vi "main(Test DQMH modules).vi"() -> ()   [LabVIEW 2018, in "Application.lvlib"] (continued)
          n6544 = Unbundle By Name(w14061) -> ("command"=w14060:string, "data"=w14059:variant)
          n6545 = call "App enquece.vi"("command data"=w14059, "command"=w14060, "queue in"=w14062) -> ("error out"=w14058:errorcluster)  [unwired: 7 in, 1 out]
        }
        n6546 = Merge Errors(w13977, w13976) -> (w13975:errorcluster)
      }
      frame "Test DRV 43A" {
        w14066 = 43 ("DUT index(0-59)")
        n6547 = disable-structure shown="LOGGING==TRUE" {
          disable-tunnel: w14071 -> [w14154 _]
          frame condition #0 (active) {
            n6548 = Empty String/Path?(string/path=w14154) -> (empty?=w14156:bool)
            n6549 = Select(t="Quece timeout", s=w14156, f=w14154) -> (s? t:f=w14153:string)
            n6550 = call "string log (SubVI).vi"("state Name"=w14153) -> ()  [unwired: 9 in, 2 out]
          }
          frame condition #1 {
          }
        }
        n6551 = Flush Queue(queue=w14072) -> (queue out=w14073:refnum<queue>)  [unwired: 1 in, 2 out]
        n6552 = Decrement(x=w14066) -> (x-1=w14070:i32)
        n6553 = Index Array(array=w14067, index=w14070) -> (element=w14068:refnum<vi>)
        n6554 = call "FGV DRV stand.vi"() -> ("Sub-Test.DCV"=w14063:bool)  [unwired: 10 in, 1 out]
        n6555 = call "FGV Driver Data.vi"("DUT index(1-60)"=w14066) -> ("DUT SC"=w14064:bool)  [unwired: 7 in, 3 out]
        n6556 = property class="ColBox"(reference=w14068, "Value"=u32 10000536 ("DRV 1")) -> ()  [unwired: 1 in, 2 out]
        n6557 = case shown="False" w14064 {
          tunnel: w14066 -> [w14084 _]
          tunnel: [w14083 w14149] -> w14065
          tunnel: w14063 -> [w14082 _]
          frame False {
            n6558 = case shown="False" w14082 {
              tunnel: w14084 -> [w14091 w14121]
              tunnel: [w14102 w14120] -> w14083
              frame False {
                w14088 = T9 {"command"="", "data"=variant} ("element")
                w14101 = T9 {"command"="", "data"=variant} ("element")
                n6559 = To Variant(anything=T3."mux10_1_channel8" ("mux10_1(x6)_encode")) -> (Variant=w14099:variant)
                n6560 = To Variant(anything=T4."demux1_10_channel8" ("demux1_10(x6)_encode")) -> (Variant=w14095:variant)
                n6561 = To Variant(anything=bool[] [TRUE, FALSE, FALSE, FALSE, FALSE, FALSE]) -> (Variant=w14110:variant)
                n6562 = Bundle By Name(cluster=w14101, "command"="MEAS.AllRelaysOFF") -> (w14109:T9)
                n6563 = Bundle By Name(cluster=w14101, "command"="MEAS.mux10-1", "data"=w14099) -> (w14092:T9)
                n6564 = Bundle By Name(cluster=w14101, "command"="MEAS.demux1-10", "data"=w14095) -> (w14093:T9)
                n6565 = Bundle By Name(cluster=w14101, "command"="MEAS.eMIC", "data"=w14110) -> (w14094:T9)
                n6566 = Build Array(w14109, w14092, w14093, w14094) -> (w14087:T9[])
                n6567 = To Variant(anything=w14091) -> (Variant=w14090:variant)
                n6568 = To Variant(anything=w14091) -> (Variant=w14089:variant)
                n6569 = Bundle By Name(cluster=w14088, "command"="MEAS.requestAC", "data"=w14090) -> (w14107:T9)
                n6570 = Bundle By Name(cluster=w14088, "command"="Apps.WaitForEvent", "data"=w14089) -> (w14103:T9)
                n6571 = Bundle By Name(cluster=w14088, "command"="Apps.UI Update 1") -> (w14104:T9)
                n6572 = Bundle By Name(cluster=w14088, "command"="WaitFor") -> (w14086:T9)
                n6573 = Build Array (concatenate)(w14087, w14086, w14107, w14103, w14104) -> (w14102:T9[])
              }
              frame True {
                w14117 = T9 {"command"="", "data"=variant} ("element")
                w14139 = T9 {"command"="", "data"=variant} ("element")
                n6574 = To Variant(anything=T3."mux10_1_channel8" ("mux10_1(x6)_encode")) -> (Variant=w14146:variant)
                n6575 = To Variant(anything=T2."mux6_1_channel1_3" ("mux6_1(3wires)_encode")) -> (Variant=w14144:variant)
                n6576 = To Variant(anything=T4."demux1_10_channel1" ("demux1_10(x6)_encode")) -> (Variant=w14140:variant)
                n6577 = To Variant(anything=bool[] [TRUE, FALSE, FALSE, FALSE, FALSE, FALSE]) -> (Variant=w14136:variant)
                n6578 = Bundle By Name(cluster=w14139, "command"="MEAS.AllRelaysOFF") -> (w14135:T9)
                n6579 = Bundle By Name(cluster=w14139, "command"="MEAS.mux10-1", "data"=w14146) -> (w14134:T9)
                n6580 = Bundle By Name(cluster=w14139, "command"="MEAS.mux6_1", "data"=w14144) -> (w14133:T9)
                n6581 = Bundle By Name(cluster=w14139, "command"="MEAS.demux1-10", "data"=w14140) -> (w14132:T9)
                n6582 = Bundle By Name(cluster=w14139, "command"="MEAS.eMIC", "data"=w14136) -> (w14131:T9)
                n6583 = Build Array(w14135, w14134, w14133, w14132, w14131) -> (w14116:T9[])
                n6584 = To Variant(anything=w14121) -> (Variant=w14119:variant)
                n6585 = To Variant(anything=w14121) -> (Variant=w14118:variant)
                n6586 = Bundle By Name(cluster=w14117, "command"="WaitFor") -> (w14115:T9)
                n6587 = Bundle By Name(cluster=w14117, "command"="MEAS.DMM dual read") -> (w14128:T9)
                n6588 = Bundle By Name(cluster=w14117, "command"="MEAS.requestAC", "data"=w14119) -> (w14127:T9)
                n6589 = Bundle By Name(cluster=w14117, "command"="Apps.WaitForEvent", "data"=w14118) -> (w14122:T9)
                n6590 = Bundle By Name(cluster=w14117, "command"="Apps.UI Update 1") -> (w14123:T9)
                n6591 = Build Array (concatenate)(w14116, w14115, w14128, w14127, w14122, w14123) -> (w14120:T9[])
              }
            }
          }
          frame True {
            n6592 = Bundle By Name(cluster=T9 {"command"="", "data"=variant} ("element"), "command"="Apps.UI Update 1") -> (w14150:T9)
            n6593 = Build Array(w14150) -> (w14149:T9[])
          }
        }
        n6594 = for {
          tunnel: w14065 -> [w14160] mode=indexing
          tunnel: w14073 -> [w14161]
          tunnel: [w14157] -> w14075 mode=indexing
          n6595 = Unbundle By Name(w14160) -> ("command"=w14159:string, "data"=w14158:variant)
          n6596 = call "App enquece.vi"("command data"=w14158, "command"=w14159, "queue in"=w14161) -> ("error out"=w14157:errorcluster)  [unwired: 7 in, 1 out]
        }
        n6597 = Merge Errors(w14076, w14075) -> (w14074:errorcluster)
      }
      frame "Test DRV 44A" {
        w14165 = 44 ("DUT index(0-59)")
        n6598 = disable-structure shown="LOGGING==TRUE" {
          disable-tunnel: w14170 -> [w14253 _]
          frame condition #0 (active) {
            n6599 = Empty String/Path?(string/path=w14253) -> (empty?=w14255:bool)
            n6600 = Select(t="Quece timeout", s=w14255, f=w14253) -> (s? t:f=w14252:string)
            n6601 = call "string log (SubVI).vi"("state Name"=w14252) -> ()  [unwired: 9 in, 2 out]
          }
          frame condition #1 {
          }
        }
        n6602 = Flush Queue(queue=w14171) -> (queue out=w14172:refnum<queue>)  [unwired: 1 in, 2 out]
        n6603 = Decrement(x=w14165) -> (x-1=w14169:i32)
        n6604 = Index Array(array=w14166, index=w14169) -> (element=w14167:refnum<vi>)
        n6605 = call "FGV DRV stand.vi"() -> ("Sub-Test.DCV"=w14162:bool)  [unwired: 10 in, 1 out]
        n6606 = call "FGV Driver Data.vi"("DUT index(1-60)"=w14165) -> ("DUT SC"=w14163:bool)  [unwired: 7 in, 3 out]
        n6607 = property class="ColBox"(reference=w14167, "Value"=u32 10000536 ("DRV 1")) -> ()  [unwired: 1 in, 2 out]
        n6608 = case shown="False" w14163 {
          tunnel: w14165 -> [w14183 _]
          tunnel: [w14182 w14248] -> w14164
          tunnel: w14162 -> [w14181 _]
          frame False {
            n6609 = case shown="False" w14181 {
              tunnel: w14183 -> [w14190 w14220]
              tunnel: [w14201 w14219] -> w14182
              frame False {
                w14187 = T9 {"command"="", "data"=variant} ("element")
                w14200 = T9 {"command"="", "data"=variant} ("element")
                n6610 = To Variant(anything=T3."mux10_1_channel8" ("mux10_1(x6)_encode")) -> (Variant=w14198:variant)
                n6611 = To Variant(anything=T4."demux1_10_channel8" ("demux1_10(x6)_encode")) -> (Variant=w14194:variant)
                n6612 = To Variant(anything=bool[] [FALSE, TRUE, FALSE, FALSE, FALSE, FALSE]) -> (Variant=w14209:variant)
                n6613 = Bundle By Name(cluster=w14200, "command"="MEAS.AllRelaysOFF") -> (w14208:T9)
                n6614 = Bundle By Name(cluster=w14200, "command"="MEAS.mux10-1", "data"=w14198) -> (w14191:T9)
                n6615 = Bundle By Name(cluster=w14200, "command"="MEAS.demux1-10", "data"=w14194) -> (w14192:T9)
                n6616 = Bundle By Name(cluster=w14200, "command"="MEAS.eMIC", "data"=w14209) -> (w14193:T9)
                n6617 = Build Array(w14208, w14191, w14192, w14193) -> (w14186:T9[])
                n6618 = To Variant(anything=w14190) -> (Variant=w14189:variant)
                n6619 = To Variant(anything=w14190) -> (Variant=w14188:variant)
                n6620 = Bundle By Name(cluster=w14187, "command"="MEAS.requestAC", "data"=w14189) -> (w14206:T9)
                n6621 = Bundle By Name(cluster=w14187, "command"="Apps.WaitForEvent", "data"=w14188) -> (w14202:T9)
                n6622 = Bundle By Name(cluster=w14187, "command"="Apps.UI Update 1") -> (w14203:T9)
                n6623 = Bundle By Name(cluster=w14187, "command"="WaitFor") -> (w14185:T9)
                n6624 = Build Array (concatenate)(w14186, w14185, w14206, w14202, w14203) -> (w14201:T9[])
              }
              frame True {
                w14216 = T9 {"command"="", "data"=variant} ("element")
                w14238 = T9 {"command"="", "data"=variant} ("element")
                n6625 = To Variant(anything=T3."mux10_1_channel8" ("mux10_1(x6)_encode")) -> (Variant=w14245:variant)
                n6626 = To Variant(anything=T2."mux6_1_channel2_3" ("mux6_1(3wires)_encode")) -> (Variant=w14243:variant)
                n6627 = To Variant(anything=T4."demux1_10_channel1" ("demux1_10(x6)_encode")) -> (Variant=w14239:variant)
                n6628 = To Variant(anything=bool[] [FALSE, TRUE, FALSE, FALSE, FALSE, FALSE]) -> (Variant=w14235:variant)
                n6629 = Bundle By Name(cluster=w14238, "command"="MEAS.AllRelaysOFF") -> (w14234:T9)
                n6630 = Bundle By Name(cluster=w14238, "command"="MEAS.mux10-1", "data"=w14245) -> (w14233:T9)
                n6631 = Bundle By Name(cluster=w14238, "command"="MEAS.mux6_1", "data"=w14243) -> (w14232:T9)
                n6632 = Bundle By Name(cluster=w14238, "command"="MEAS.demux1-10", "data"=w14239) -> (w14231:T9)
                n6633 = Bundle By Name(cluster=w14238, "command"="MEAS.eMIC", "data"=w14235) -> (w14230:T9)
                n6634 = Build Array(w14234, w14233, w14232, w14231, w14230) -> (w14215:T9[])
                n6635 = To Variant(anything=w14220) -> (Variant=w14218:variant)
                n6636 = To Variant(anything=w14220) -> (Variant=w14217:variant)
                n6637 = Bundle By Name(cluster=w14216, "command"="WaitFor") -> (w14214:T9)
                n6638 = Bundle By Name(cluster=w14216, "command"="MEAS.DMM dual read") -> (w14227:T9)
                n6639 = Bundle By Name(cluster=w14216, "command"="MEAS.requestAC", "data"=w14218) -> (w14226:T9)
                n6640 = Bundle By Name(cluster=w14216, "command"="Apps.WaitForEvent", "data"=w14217) -> (w14221:T9)
                n6641 = Bundle By Name(cluster=w14216, "command"="Apps.UI Update 1") -> (w14222:T9)
                n6642 = Build Array (concatenate)(w14215, w14214, w14227, w14226, w14221, w14222) -> (w14219:T9[])
              }
            }
          }
          frame True {
            n6643 = Bundle By Name(cluster=T9 {"command"="", "data"=variant} ("element"), "command"="Apps.UI Update 1") -> (w14249:T9)
            n6644 = Build Array(w14249) -> (w14248:T9[])
          }
        }
        n6645 = for {
          tunnel: w14164 -> [w14259] mode=indexing
          tunnel: w14172 -> [w14260]
          tunnel: [w14256] -> w14174 mode=indexing
          n6646 = Unbundle By Name(w14259) -> ("command"=w14258:string, "data"=w14257:variant)
          n6647 = call "App enquece.vi"("command data"=w14257, "command"=w14258, "queue in"=w14260) -> ("error out"=w14256:errorcluster)  [unwired: 7 in, 1 out]
        }
        n6648 = Merge Errors(w14175, w14174) -> (w14173:errorcluster)
      }
      frame "Test DRV 45A" {
        w14264 = 45 ("DUT index(0-59)")
        n6649 = disable-structure shown="LOGGING==TRUE" {
          disable-tunnel: w14269 -> [w14352 _]
          frame condition #0 (active) {
            n6650 = Empty String/Path?(string/path=w14352) -> (empty?=w14354:bool)
            n6651 = Select(t="Quece timeout", s=w14354, f=w14352) -> (s? t:f=w14351:string)
            n6652 = call "string log (SubVI).vi"("state Name"=w14351) -> ()  [unwired: 9 in, 2 out]
          }
          frame condition #1 {
          }
        }
        n6653 = Flush Queue(queue=w14270) -> (queue out=w14271:refnum<queue>)  [unwired: 1 in, 2 out]
        n6654 = Decrement(x=w14264) -> (x-1=w14268:i32)
        n6655 = Index Array(array=w14265, index=w14268) -> (element=w14266:refnum<vi>)
        n6656 = call "FGV DRV stand.vi"() -> ("Sub-Test.DCV"=w14261:bool)  [unwired: 10 in, 1 out]
        n6657 = call "FGV Driver Data.vi"("DUT index(1-60)"=w14264) -> ("DUT SC"=w14262:bool)  [unwired: 7 in, 3 out]
        n6658 = property class="ColBox"(reference=w14266, "Value"=u32 10000536 ("DRV 1")) -> ()  [unwired: 1 in, 2 out]
        n6659 = case shown="False" w14262 {
          tunnel: w14264 -> [w14282 _]
          tunnel: [w14281 w14347] -> w14263
          tunnel: w14261 -> [w14280 _]
          frame False {
            n6660 = case shown="True" w14280 {
              tunnel: w14282 -> [w14289 w14319]
              tunnel: [w14300 w14318] -> w14281
              frame False {
                w14286 = T9 {"command"="", "data"=variant} ("element")
                w14299 = T9 {"command"="", "data"=variant} ("element")
                n6661 = To Variant(anything=T3."mux10_1_channel8" ("mux10_1(x6)_encode")) -> (Variant=w14297:variant)
                n6662 = To Variant(anything=T4."demux1_10_channel8" ("demux1_10(x6)_encode")) -> (Variant=w14293:variant)
                n6663 = To Variant(anything=bool[] [FALSE, FALSE, TRUE, FALSE, FALSE, FALSE]) -> (Variant=w14308:variant)
                n6664 = Bundle By Name(cluster=w14299, "command"="MEAS.AllRelaysOFF") -> (w14307:T9)
                n6665 = Bundle By Name(cluster=w14299, "command"="MEAS.mux10-1", "data"=w14297) -> (w14290:T9)
                n6666 = Bundle By Name(cluster=w14299, "command"="MEAS.demux1-10", "data"=w14293) -> (w14291:T9)
                n6667 = Bundle By Name(cluster=w14299, "command"="MEAS.eMIC", "data"=w14308) -> (w14292:T9)
                n6668 = Build Array(w14307, w14290, w14291, w14292) -> (w14285:T9[])
                n6669 = To Variant(anything=w14289) -> (Variant=w14288:variant)
                n6670 = To Variant(anything=w14289) -> (Variant=w14287:variant)
                n6671 = Bundle By Name(cluster=w14286, "command"="MEAS.requestAC", "data"=w14288) -> (w14305:T9)
                n6672 = Bundle By Name(cluster=w14286, "command"="Apps.WaitForEvent", "data"=w14287) -> (w14301:T9)
                n6673 = Bundle By Name(cluster=w14286, "command"="Apps.UI Update 1") -> (w14302:T9)
                n6674 = Bundle By Name(cluster=w14286, "command"="WaitFor") -> (w14284:T9)
                n6675 = Build Array (concatenate)(w14285, w14284, w14305, w14301, w14302) -> (w14300:T9[])
              }
              frame True {
                w14315 = T9 {"command"="", "data"=variant} ("element")
                w14337 = T9 {"command"="", "data"=variant} ("element")
                n6676 = To Variant(anything=T3."mux10_1_channel8" ("mux10_1(x6)_encode")) -> (Variant=w14344:variant)
                n6677 = To Variant(anything=T2."mux6_1_channel3_3" ("mux6_1(3wires)_encode")) -> (Variant=w14342:variant)
                n6678 = To Variant(anything=T4."demux1_10_channel1" ("demux1_10(x6)_encode")) -> (Variant=w14338:variant)
                n6679 = To Variant(anything=bool[] [FALSE, FALSE, TRUE, FALSE, FALSE, FALSE]) -> (Variant=w14334:variant)
                n6680 = Bundle By Name(cluster=w14337, "command"="MEAS.AllRelaysOFF") -> (w14333:T9)
                n6681 = Bundle By Name(cluster=w14337, "command"="MEAS.mux10-1", "data"=w14344) -> (w14332:T9)
                n6682 = Bundle By Name(cluster=w14337, "command"="MEAS.mux6_1", "data"=w14342) -> (w14331:T9)
                n6683 = Bundle By Name(cluster=w14337, "command"="MEAS.demux1-10", "data"=w14338) -> (w14330:T9)
                n6684 = Bundle By Name(cluster=w14337, "command"="MEAS.eMIC", "data"=w14334) -> (w14329:T9)
                n6685 = Build Array(w14333, w14332, w14331, w14330, w14329) -> (w14314:T9[])
                n6686 = To Variant(anything=w14319) -> (Variant=w14317:variant)
                n6687 = To Variant(anything=w14319) -> (Variant=w14316:variant)
                n6688 = Bundle By Name(cluster=w14315, "command"="WaitFor") -> (w14313:T9)
                n6689 = Bundle By Name(cluster=w14315, "command"="MEAS.DMM dual read") -> (w14326:T9)
                n6690 = Bundle By Name(cluster=w14315, "command"="MEAS.requestAC", "data"=w14317) -> (w14325:T9)
                n6691 = Bundle By Name(cluster=w14315, "command"="Apps.WaitForEvent", "data"=w14316) -> (w14320:T9)
                n6692 = Bundle By Name(cluster=w14315, "command"="Apps.UI Update 1") -> (w14321:T9)
                n6693 = Build Array (concatenate)(w14314, w14313, w14326, w14325, w14320, w14321) -> (w14318:T9[])
              }
            }
          }
          frame True {
            n6694 = Bundle By Name(cluster=T9 {"command"="", "data"=variant} ("element"), "command"="Apps.UI Update 1") -> (w14348:T9)
            n6695 = Build Array(w14348) -> (w14347:T9[])
          }
        }
        n6696 = for {
          tunnel: w14263 -> [w14358] mode=indexing
          tunnel: w14271 -> [w14359]
          tunnel: [w14355] -> w14273 mode=indexing
          n6697 = Unbundle By Name(w14358) -> ("command"=w14357:string, "data"=w14356:variant)
          n6698 = call "App enquece.vi"("command data"=w14356, "command"=w14357, "queue in"=w14359) -> ("error out"=w14355:errorcluster)  [unwired: 7 in, 1 out]
        }
        n6699 = Merge Errors(w14274, w14273) -> (w14272:errorcluster)
      }
      frame "Test DRV 46A" {
        w14363 = 46 ("DUT index(0-59)")
        n6700 = disable-structure shown="LOGGING==TRUE" {
          disable-tunnel: w14368 -> [w14451 _]
          frame condition #0 (active) {
            n6701 = Empty String/Path?(string/path=w14451) -> (empty?=w14453:bool)
            n6702 = Select(t="Quece timeout", s=w14453, f=w14451) -> (s? t:f=w14450:string)
            n6703 = call "string log (SubVI).vi"("state Name"=w14450) -> ()  [unwired: 9 in, 2 out]
          }
          frame condition #1 {
          }
        }
        n6704 = Flush Queue(queue=w14369) -> (queue out=w14370:refnum<queue>)  [unwired: 1 in, 2 out]
        n6705 = Decrement(x=w14363) -> (x-1=w14367:i32)
        n6706 = Index Array(array=w14364, index=w14367) -> (element=w14365:refnum<vi>)
        n6707 = call "FGV DRV stand.vi"() -> ("Sub-Test.DCV"=w14360:bool)  [unwired: 10 in, 1 out]
        n6708 = call "FGV Driver Data.vi"("DUT index(1-60)"=w14363) -> ("DUT SC"=w14361:bool)  [unwired: 7 in, 3 out]
        n6709 = property class="ColBox"(reference=w14365, "Value"=u32 10000536 ("DRV 1")) -> ()  [unwired: 1 in, 2 out]
        n6710 = case shown="False" w14361 {
          tunnel: w14363 -> [w14381 _]
          tunnel: [w14380 w14446] -> w14362
          tunnel: w14360 -> [w14379 _]
          frame False {
            n6711 = case shown="True" w14379 {
              tunnel: w14381 -> [w14388 w14418]
              tunnel: [w14399 w14417] -> w14380
              frame False {
                w14385 = T9 {"command"="", "data"=variant} ("element")
                w14398 = T9 {"command"="", "data"=variant} ("element")
                n6712 = To Variant(anything=T3."mux10_1_channel8" ("mux10_1(x6)_encode")) -> (Variant=w14396:variant)
                n6713 = To Variant(anything=T4."demux1_10_channel8" ("demux1_10(x6)_encode")) -> (Variant=w14392:variant)
                n6714 = To Variant(anything=bool[] [FALSE, FALSE, FALSE, TRUE, FALSE, FALSE]) -> (Variant=w14407:variant)
                n6715 = Bundle By Name(cluster=w14398, "command"="MEAS.AllRelaysOFF") -> (w14406:T9)
                n6716 = Bundle By Name(cluster=w14398, "command"="MEAS.mux10-1", "data"=w14396) -> (w14389:T9)
                n6717 = Bundle By Name(cluster=w14398, "command"="MEAS.demux1-10", "data"=w14392) -> (w14390:T9)
                n6718 = Bundle By Name(cluster=w14398, "command"="MEAS.eMIC", "data"=w14407) -> (w14391:T9)
                n6719 = Build Array(w14406, w14389, w14390, w14391) -> (w14384:T9[])
                n6720 = To Variant(anything=w14388) -> (Variant=w14387:variant)
                n6721 = To Variant(anything=w14388) -> (Variant=w14386:variant)
                n6722 = Bundle By Name(cluster=w14385, "command"="MEAS.requestAC", "data"=w14387) -> (w14404:T9)
                n6723 = Bundle By Name(cluster=w14385, "command"="Apps.WaitForEvent", "data"=w14386) -> (w14400:T9)
                n6724 = Bundle By Name(cluster=w14385, "command"="Apps.UI Update 1") -> (w14401:T9)
                n6725 = Bundle By Name(cluster=w14385, "command"="WaitFor") -> (w14383:T9)
                n6726 = Build Array (concatenate)(w14384, w14383, w14404, w14400, w14401) -> (w14399:T9[])
              }
              frame True {
                w14414 = T9 {"command"="", "data"=variant} ("element")
                w14436 = T9 {"command"="", "data"=variant} ("element")
                n6727 = To Variant(anything=T3."mux10_1_channel8" ("mux10_1(x6)_encode")) -> (Variant=w14443:variant)
                n6728 = To Variant(anything=T2."mux6_1_channel4_3" ("mux6_1(3wires)_encode")) -> (Variant=w14441:variant)
                n6729 = To Variant(anything=T4."demux1_10_channel1" ("demux1_10(x6)_encode")) -> (Variant=w14437:variant)
                n6730 = To Variant(anything=bool[] [FALSE, FALSE, FALSE, TRUE, FALSE, FALSE]) -> (Variant=w14433:variant)
                n6731 = Bundle By Name(cluster=w14436, "command"="MEAS.AllRelaysOFF") -> (w14432:T9)
                n6732 = Bundle By Name(cluster=w14436, "command"="MEAS.mux10-1", "data"=w14443) -> (w14431:T9)
                n6733 = Bundle By Name(cluster=w14436, "command"="MEAS.mux6_1", "data"=w14441) -> (w14430:T9)
                n6734 = Bundle By Name(cluster=w14436, "command"="MEAS.demux1-10", "data"=w14437) -> (w14429:T9)
                n6735 = Bundle By Name(cluster=w14436, "command"="MEAS.eMIC", "data"=w14433) -> (w14428:T9)
                n6736 = Build Array(w14432, w14431, w14430, w14429, w14428) -> (w14413:T9[])
                n6737 = To Variant(anything=w14418) -> (Variant=w14416:variant)
                n6738 = To Variant(anything=w14418) -> (Variant=w14415:variant)
                n6739 = Bundle By Name(cluster=w14414, "command"="WaitFor") -> (w14412:T9)
                n6740 = Bundle By Name(cluster=w14414, "command"="MEAS.DMM dual read") -> (w14425:T9)
                n6741 = Bundle By Name(cluster=w14414, "command"="MEAS.requestAC", "data"=w14416) -> (w14424:T9)
                n6742 = Bundle By Name(cluster=w14414, "command"="Apps.WaitForEvent", "data"=w14415) -> (w14419:T9)
                n6743 = Bundle By Name(cluster=w14414, "command"="Apps.UI Update 1") -> (w14420:T9)
                n6744 = Build Array (concatenate)(w14413, w14412, w14425, w14424, w14419, w14420) -> (w14417:T9[])
              }
            }
          }
          frame True {
            n6745 = Bundle By Name(cluster=T9 {"command"="", "data"=variant} ("element"), "command"="Apps.UI Update 1") -> (w14447:T9)
            n6746 = Build Array(w14447) -> (w14446:T9[])
          }
        }
        n6747 = for {
          tunnel: w14362 -> [w14457] mode=indexing
          tunnel: w14370 -> [w14458]
          tunnel: [w14454] -> w14372 mode=indexing
          n6748 = Unbundle By Name(w14457) -> ("command"=w14456:string, "data"=w14455:variant)
          n6749 = call "App enquece.vi"("command data"=w14455, "command"=w14456, "queue in"=w14458) -> ("error out"=w14454:errorcluster)  [unwired: 7 in, 1 out]
        }
        n6750 = Merge Errors(w14373, w14372) -> (w14371:errorcluster)
      }
      frame "Test DRV 47A" {
        w14462 = 47 ("DUT index(0-59)")
        n6751 = disable-structure shown="LOGGING==TRUE" {
          disable-tunnel: w14467 -> [w14550 _]
          frame condition #0 (active) {
            n6752 = Empty String/Path?(string/path=w14550) -> (empty?=w14552:bool)
            n6753 = Select(t="Quece timeout", s=w14552, f=w14550) -> (s? t:f=w14549:string)
            n6754 = call "string log (SubVI).vi"("state Name"=w14549) -> ()  [unwired: 9 in, 2 out]
          }
          frame condition #1 {
          }
        }
        n6755 = Flush Queue(queue=w14468) -> (queue out=w14469:refnum<queue>)  [unwired: 1 in, 2 out]
        n6756 = Decrement(x=w14462) -> (x-1=w14466:i32)
        n6757 = Index Array(array=w14463, index=w14466) -> (element=w14464:refnum<vi>)
        n6758 = call "FGV DRV stand.vi"() -> ("Sub-Test.DCV"=w14459:bool)  [unwired: 10 in, 1 out]
        n6759 = call "FGV Driver Data.vi"("DUT index(1-60)"=w14462) -> ("DUT SC"=w14460:bool)  [unwired: 7 in, 3 out]
        n6760 = property class="ColBox"(reference=w14464, "Value"=u32 10000536 ("DRV 1")) -> ()  [unwired: 1 in, 2 out]
        n6761 = case shown="False" w14460 {
          tunnel: w14462 -> [w14480 _]
          tunnel: [w14479 w14545] -> w14461
          tunnel: w14459 -> [w14478 _]
          frame False {
            n6762 = case shown="False" w14478 {
              tunnel: w14480 -> [w14487 w14517]
              tunnel: [w14498 w14516] -> w14479
              frame False {
                w14484 = T9 {"command"="", "data"=variant} ("element")
                w14497 = T9 {"command"="", "data"=variant} ("element")
                n6763 = To Variant(anything=T3."mux10_1_channel8" ("mux10_1(x6)_encode")) -> (Variant=w14495:variant)
                n6764 = To Variant(anything=T4."demux1_10_channel8" ("demux1_10(x6)_encode")) -> (Variant=w14491:variant)
                n6765 = To Variant(anything=bool[] [FALSE, FALSE, FALSE, FALSE, TRUE, FALSE]) -> (Variant=w14506:variant)
                n6766 = Bundle By Name(cluster=w14497, "command"="MEAS.AllRelaysOFF") -> (w14505:T9)
                n6767 = Bundle By Name(cluster=w14497, "command"="MEAS.mux10-1", "data"=w14495) -> (w14488:T9)
                n6768 = Bundle By Name(cluster=w14497, "command"="MEAS.demux1-10", "data"=w14491) -> (w14489:T9)
                n6769 = Bundle By Name(cluster=w14497, "command"="MEAS.eMIC", "data"=w14506) -> (w14490:T9)
                n6770 = Build Array(w14505, w14488, w14489, w14490) -> (w14483:T9[])
                n6771 = To Variant(anything=w14487) -> (Variant=w14486:variant)
                n6772 = To Variant(anything=w14487) -> (Variant=w14485:variant)
                n6773 = Bundle By Name(cluster=w14484, "command"="MEAS.requestAC", "data"=w14486) -> (w14503:T9)
                n6774 = Bundle By Name(cluster=w14484, "command"="Apps.WaitForEvent", "data"=w14485) -> (w14499:T9)
                n6775 = Bundle By Name(cluster=w14484, "command"="Apps.UI Update 1") -> (w14500:T9)
                n6776 = Bundle By Name(cluster=w14484, "command"="WaitFor") -> (w14482:T9)
                n6777 = Build Array (concatenate)(w14483, w14482, w14503, w14499, w14500) -> (w14498:T9[])
              }
              frame True {
                w14513 = T9 {"command"="", "data"=variant} ("element")
                w14535 = T9 {"command"="", "data"=variant} ("element")
                n6778 = To Variant(anything=T3."mux10_1_channel8" ("mux10_1(x6)_encode")) -> (Variant=w14542:variant)
                n6779 = To Variant(anything=T2."mux6_1_channel5_3" ("mux6_1(3wires)_encode")) -> (Variant=w14540:variant)
                n6780 = To Variant(anything=T4."demux1_10_channel1" ("demux1_10(x6)_encode")) -> (Variant=w14536:variant)
                n6781 = To Variant(anything=bool[] [FALSE, FALSE, FALSE, FALSE, TRUE, FALSE]) -> (Variant=w14532:variant)
                n6782 = Bundle By Name(cluster=w14535, "command"="MEAS.AllRelaysOFF") -> (w14531:T9)
                n6783 = Bundle By Name(cluster=w14535, "command"="MEAS.mux10-1", "data"=w14542) -> (w14530:T9)
                n6784 = Bundle By Name(cluster=w14535, "command"="MEAS.mux6_1", "data"=w14540) -> (w14529:T9)
                n6785 = Bundle By Name(cluster=w14535, "command"="MEAS.demux1-10", "data"=w14536) -> (w14528:T9)
                n6786 = Bundle By Name(cluster=w14535, "command"="MEAS.eMIC", "data"=w14532) -> (w14527:T9)
                n6787 = Build Array(w14531, w14530, w14529, w14528, w14527) -> (w14512:T9[])
                n6788 = To Variant(anything=w14517) -> (Variant=w14515:variant)
                n6789 = To Variant(anything=w14517) -> (Variant=w14514:variant)
                n6790 = Bundle By Name(cluster=w14513, "command"="WaitFor") -> (w14511:T9)
                n6791 = Bundle By Name(cluster=w14513, "command"="MEAS.DMM dual read") -> (w14524:T9)
                n6792 = Bundle By Name(cluster=w14513, "command"="MEAS.requestAC", "data"=w14515) -> (w14523:T9)
                n6793 = Bundle By Name(cluster=w14513, "command"="Apps.WaitForEvent", "data"=w14514) -> (w14518:T9)
                n6794 = Bundle By Name(cluster=w14513, "command"="Apps.UI Update 1") -> (w14519:T9)
                n6795 = Build Array (concatenate)(w14512, w14511, w14524, w14523, w14518, w14519) -> (w14516:T9[])
              }
            }
          }
          frame True {
            n6796 = Bundle By Name(cluster=T9 {"command"="", "data"=variant} ("element"), "command"="Apps.UI Update 1") -> (w14546:T9)
            n6797 = Build Array(w14546) -> (w14545:T9[])
          }
        }
        n6798 = for {
          tunnel: w14461 -> [w14556] mode=indexing
          tunnel: w14469 -> [w14557]
          tunnel: [w14553] -> w14471 mode=indexing
          n6799 = Unbundle By Name(w14556) -> ("command"=w14555:string, "data"=w14554:variant)
          n6800 = call "App enquece.vi"("command data"=w14554, "command"=w14555, "queue in"=w14557) -> ("error out"=w14553:errorcluster)  [unwired: 7 in, 1 out]
        }
        n6801 = Merge Errors(w14472, w14471) -> (w14470:errorcluster)
      }
      frame "Test DRV 48A" {
        w14561 = 48 ("DUT index(0-59)")
        n6802 = disable-structure shown="LOGGING==TRUE" {
          disable-tunnel: w14566 -> [w14649 _]
          frame condition #0 (active) {
            n6803 = Empty String/Path?(string/path=w14649) -> (empty?=w14651:bool)
            n6804 = Select(t="Quece timeout", s=w14651, f=w14649) -> (s? t:f=w14648:string)
            n6805 = call "string log (SubVI).vi"("state Name"=w14648) -> ()  [unwired: 9 in, 2 out]
          }
          frame condition #1 {
          }
        }
        n6806 = Flush Queue(queue=w14567) -> (queue out=w14568:refnum<queue>)  [unwired: 1 in, 2 out]
        n6807 = Decrement(x=w14561) -> (x-1=w14565:i32)
        n6808 = Index Array(array=w14562, index=w14565) -> (element=w14563:refnum<vi>)
        n6809 = call "FGV DRV stand.vi"() -> ("Sub-Test.DCV"=w14558:bool)  [unwired: 10 in, 1 out]
        n6810 = call "FGV Driver Data.vi"("DUT index(1-60)"=w14561) -> ("DUT SC"=w14559:bool)  [unwired: 7 in, 3 out]
        n6811 = property class="ColBox"(reference=w14563, "Value"=u32 10000536 ("DRV 1")) -> ()  [unwired: 1 in, 2 out]
        n6812 = case shown="False" w14559 {
          tunnel: w14561 -> [w14579 _]
          tunnel: [w14578 w14644] -> w14560
          tunnel: w14558 -> [w14577 _]
          frame False {
            n6813 = case shown="True" w14577 {
              tunnel: w14579 -> [w14586 w14616]
              tunnel: [w14597 w14615] -> w14578
              frame False {
                w14583 = T9 {"command"="", "data"=variant} ("element")
                w14596 = T9 {"command"="", "data"=variant} ("element")
                n6814 = To Variant(anything=T3."mux10_1_channel8" ("mux10_1(x6)_encode")) -> (Variant=w14594:variant)
                n6815 = To Variant(anything=T4."demux1_10_channel8" ("demux1_10(x6)_encode")) -> (Variant=w14590:variant)
                n6816 = To Variant(anything=bool[] [FALSE, FALSE, FALSE, FALSE, FALSE, TRUE]) -> (Variant=w14605:variant)
                n6817 = Bundle By Name(cluster=w14596, "command"="MEAS.AllRelaysOFF") -> (w14604:T9)
                n6818 = Bundle By Name(cluster=w14596, "command"="MEAS.mux10-1", "data"=w14594) -> (w14587:T9)
                n6819 = Bundle By Name(cluster=w14596, "command"="MEAS.demux1-10", "data"=w14590) -> (w14588:T9)
                n6820 = Bundle By Name(cluster=w14596, "command"="MEAS.eMIC", "data"=w14605) -> (w14589:T9)
                n6821 = Build Array(w14604, w14587, w14588, w14589) -> (w14582:T9[])
                n6822 = To Variant(anything=w14586) -> (Variant=w14585:variant)
                n6823 = To Variant(anything=w14586) -> (Variant=w14584:variant)
                n6824 = Bundle By Name(cluster=w14583, "command"="MEAS.requestAC", "data"=w14585) -> (w14602:T9)
                n6825 = Bundle By Name(cluster=w14583, "command"="Apps.WaitForEvent", "data"=w14584) -> (w14598:T9)
                n6826 = Bundle By Name(cluster=w14583, "command"="Apps.UI Update 1") -> (w14599:T9)
                n6827 = Bundle By Name(cluster=w14583, "command"="WaitFor") -> (w14581:T9)
                n6828 = Build Array (concatenate)(w14582, w14581, w14602, w14598, w14599) -> (w14597:T9[])
              }
              frame True {
                w14612 = T9 {"command"="", "data"=variant} ("element")
                w14634 = T9 {"command"="", "data"=variant} ("element")
                n6829 = To Variant(anything=T3."mux10_1_channel8" ("mux10_1(x6)_encode")) -> (Variant=w14641:variant)
                n6830 = To Variant(anything=T2."mux6_1_channel6_3" ("mux6_1(3wires)_encode")) -> (Variant=w14639:variant)
                n6831 = To Variant(anything=T4."demux1_10_channel1" ("demux1_10(x6)_encode")) -> (Variant=w14635:variant)
                n6832 = To Variant(anything=bool[] [FALSE, FALSE, FALSE, FALSE, FALSE, TRUE]) -> (Variant=w14631:variant)
                n6833 = Bundle By Name(cluster=w14634, "command"="MEAS.AllRelaysOFF") -> (w14630:T9)
                n6834 = Bundle By Name(cluster=w14634, "command"="MEAS.mux10-1", "data"=w14641) -> (w14629:T9)
                n6835 = Bundle By Name(cluster=w14634, "command"="MEAS.mux6_1", "data"=w14639) -> (w14628:T9)
                n6836 = Bundle By Name(cluster=w14634, "command"="MEAS.demux1-10", "data"=w14635) -> (w14627:T9)
                n6837 = Bundle By Name(cluster=w14634, "command"="MEAS.eMIC", "data"=w14631) -> (w14626:T9)
                n6838 = Build Array(w14630, w14629, w14628, w14627, w14626) -> (w14611:T9[])
                n6839 = To Variant(anything=w14616) -> (Variant=w14614:variant)
                n6840 = To Variant(anything=w14616) -> (Variant=w14613:variant)
                n6841 = Bundle By Name(cluster=w14612, "command"="WaitFor") -> (w14610:T9)
                n6842 = Bundle By Name(cluster=w14612, "command"="MEAS.DMM dual read") -> (w14623:T9)
                n6843 = Bundle By Name(cluster=w14612, "command"="MEAS.requestAC", "data"=w14614) -> (w14622:T9)
                n6844 = Bundle By Name(cluster=w14612, "command"="Apps.WaitForEvent", "data"=w14613) -> (w14617:T9)
                n6845 = Bundle By Name(cluster=w14612, "command"="Apps.UI Update 1") -> (w14618:T9)
                n6846 = Build Array (concatenate)(w14611, w14610, w14623, w14622, w14617, w14618) -> (w14615:T9[])
              }
            }
          }
          frame True {
            n6847 = Bundle By Name(cluster=T9 {"command"="", "data"=variant} ("element"), "command"="Apps.UI Update 1") -> (w14645:T9)
            n6848 = Build Array(w14645) -> (w14644:T9[])
          }
        }
        n6849 = for {
          tunnel: w14560 -> [w14655] mode=indexing
          tunnel: w14568 -> [w14656]
          tunnel: [w14652] -> w14570 mode=indexing
          n6850 = Unbundle By Name(w14655) -> ("command"=w14654:string, "data"=w14653:variant)
          n6851 = call "App enquece.vi"("command data"=w14653, "command"=w14654, "queue in"=w14656) -> ("error out"=w14652:errorcluster)  [unwired: 7 in, 1 out]
        }
        n6852 = Merge Errors(w14571, w14570) -> (w14569:errorcluster)
      }
      frame "Test DRV 49A" {
        w14660 = 49 ("DUT index(0-59)")
        n6853 = disable-structure shown="LOGGING==TRUE" {
          disable-tunnel: w14665 -> [w14748 _]
          frame condition #0 (active) {
            n6854 = Empty String/Path?(string/path=w14748) -> (empty?=w14750:bool)
            n6855 = Select(t="Quece timeout", s=w14750, f=w14748) -> (s? t:f=w14747:string)
            n6856 = call "string log (SubVI).vi"("state Name"=w14747) -> ()  [unwired: 9 in, 2 out]
          }
          frame condition #1 {
          }
        }
        n6857 = Flush Queue(queue=w14666) -> (queue out=w14667:refnum<queue>)  [unwired: 1 in, 2 out]
        n6858 = Decrement(x=w14660) -> (x-1=w14664:i32)
        n6859 = Index Array(array=w14661, index=w14664) -> (element=w14662:refnum<vi>)
        n6860 = call "FGV DRV stand.vi"() -> ("Sub-Test.DCV"=w14657:bool)  [unwired: 10 in, 1 out]
        n6861 = call "FGV Driver Data.vi"("DUT index(1-60)"=w14660) -> ("DUT SC"=w14658:bool)  [unwired: 7 in, 3 out]
        n6862 = property class="ColBox"(reference=w14662, "Value"=u32 10000536 ("DRV 1")) -> ()  [unwired: 1 in, 2 out]
        n6863 = case shown="False" w14658 {
          tunnel: w14660 -> [w14678 _]
          tunnel: [w14677 w14743] -> w14659
          tunnel: w14657 -> [w14676 _]
          frame False {
            n6864 = case shown="False" w14676 {
              tunnel: w14678 -> [w14685 w14715]
              tunnel: [w14696 w14714] -> w14677
              frame False {
                w14682 = T9 {"command"="", "data"=variant} ("element")
                w14695 = T9 {"command"="", "data"=variant} ("element")
                n6865 = To Variant(anything=T3."mux10_1_channel9" ("mux10_1(x6)_encode")) -> (Variant=w14693:variant)
                n6866 = To Variant(anything=T4."demux1_10_channel9" ("demux1_10(x6)_encode")) -> (Variant=w14689:variant)
                n6867 = To Variant(anything=bool[] [TRUE, FALSE, FALSE, FALSE, FALSE, FALSE]) -> (Variant=w14704:variant)
                n6868 = Bundle By Name(cluster=w14695, "command"="MEAS.AllRelaysOFF") -> (w14703:T9)
                n6869 = Bundle By Name(cluster=w14695, "command"="MEAS.mux10-1", "data"=w14693) -> (w14686:T9)
                n6870 = Bundle By Name(cluster=w14695, "command"="MEAS.demux1-10", "data"=w14689) -> (w14687:T9)
                n6871 = Bundle By Name(cluster=w14695, "command"="MEAS.eMIC", "data"=w14704) -> (w14688:T9)
                n6872 = Build Array(w14703, w14686, w14687, w14688) -> (w14681:T9[])
                n6873 = To Variant(anything=w14685) -> (Variant=w14684:variant)
                n6874 = To Variant(anything=w14685) -> (Variant=w14683:variant)
                n6875 = Bundle By Name(cluster=w14682, "command"="MEAS.requestAC", "data"=w14684) -> (w14701:T9)
                n6876 = Bundle By Name(cluster=w14682, "command"="Apps.WaitForEvent", "data"=w14683) -> (w14697:T9)
                n6877 = Bundle By Name(cluster=w14682, "command"="Apps.UI Update 1") -> (w14698:T9)
                n6878 = Bundle By Name(cluster=w14682, "command"="WaitFor") -> (w14680:T9)
                n6879 = Build Array (concatenate)(w14681, w14680, w14701, w14697, w14698) -> (w14696:T9[])
              }
              frame True {
                w14711 = T9 {"command"="", "data"=variant} ("element")
                w14733 = T9 {"command"="", "data"=variant} ("element")
                n6880 = To Variant(anything=T3."mux10_1_channel9" ("mux10_1(x6)_encode")) -> (Variant=w14740:variant)
                n6881 = To Variant(anything=T2."mux6_1_channel1_3" ("mux6_1(3wires)_encode")) -> (Variant=w14738:variant)
                n6882 = To Variant(anything=T4."demux1_10_channel9" ("demux1_10(x6)_encode")) -> (Variant=w14734:variant)
                n6883 = To Variant(anything=bool[] [TRUE, FALSE, FALSE, FALSE, FALSE, FALSE]) -> (Variant=w14730:variant)
                n6884 = Bundle By Name(cluster=w14733, "command"="MEAS.AllRelaysOFF") -> (w14729:T9)
                n6885 = Bundle By Name(cluster=w14733, "command"="MEAS.mux10-1", "data"=w14740) -> (w14728:T9)
                n6886 = Bundle By Name(cluster=w14733, "command"="MEAS.mux6_1", "data"=w14738) -> (w14727:T9)
                n6887 = Bundle By Name(cluster=w14733, "command"="MEAS.demux1-10", "data"=w14734) -> (w14726:T9)
                n6888 = Bundle By Name(cluster=w14733, "command"="MEAS.eMIC", "data"=w14730) -> (w14725:T9)
                n6889 = Build Array(w14729, w14728, w14727, w14726, w14725) -> (w14710:T9[])
                n6890 = To Variant(anything=w14715) -> (Variant=w14713:variant)
                n6891 = To Variant(anything=w14715) -> (Variant=w14712:variant)
                n6892 = Bundle By Name(cluster=w14711, "command"="WaitFor") -> (w14709:T9)
                n6893 = Bundle By Name(cluster=w14711, "command"="MEAS.DMM dual read") -> (w14722:T9)
                n6894 = Bundle By Name(cluster=w14711, "command"="MEAS.requestAC", "data"=w14713) -> (w14721:T9)
                n6895 = Bundle By Name(cluster=w14711, "command"="Apps.WaitForEvent", "data"=w14712) -> (w14716:T9)
                n6896 = Bundle By Name(cluster=w14711, "command"="Apps.UI Update 1") -> (w14717:T9)
                n6897 = Build Array (concatenate)(w14710, w14709, w14722, w14721, w14716, w14717) -> (w14714:T9[])
              }
            }
          }
          frame True {
            n6898 = Bundle By Name(cluster=T9 {"command"="", "data"=variant} ("element"), "command"="Apps.UI Update 1") -> (w14744:T9)
            n6899 = Build Array(w14744) -> (w14743:T9[])
          }
        }
        n6900 = for {
          tunnel: w14659 -> [w14754] mode=indexing
          tunnel: w14667 -> [w14755]
          tunnel: [w14751] -> w14669 mode=indexing
          n6901 = Unbundle By Name(w14754) -> ("command"=w14753:string, "data"=w14752:variant)
          n6902 = call "App enquece.vi"("command data"=w14752, "command"=w14753, "queue in"=w14755) -> ("error out"=w14751:errorcluster)  [unwired: 7 in, 1 out]
        }
        n6903 = Merge Errors(w14670, w14669) -> (w14668:errorcluster)
      }
      frame "Test DRV 50A" {
        w14759 = 50 ("DUT index(0-59)")
        n6904 = disable-structure shown="LOGGING==TRUE" {
          disable-tunnel: w14764 -> [w14847 _]
          frame condition #0 (active) {
            n6905 = Empty String/Path?(string/path=w14847) -> (empty?=w14849:bool)
            n6906 = Select(t="Quece timeout", s=w14849, f=w14847) -> (s? t:f=w14846:string)
            n6907 = call "string log (SubVI).vi"("state Name"=w14846) -> ()  [unwired: 9 in, 2 out]
          }
          frame condition #1 {
          }
        }
        n6908 = Flush Queue(queue=w14765) -> (queue out=w14766:refnum<queue>)  [unwired: 1 in, 2 out]
        n6909 = Decrement(x=w14759) -> (x-1=w14763:i32)
        n6910 = Index Array(array=w14760, index=w14763) -> (element=w14761:refnum<vi>)
        n6911 = call "FGV DRV stand.vi"() -> ("Sub-Test.DCV"=w14756:bool)  [unwired: 10 in, 1 out]
        n6912 = call "FGV Driver Data.vi"("DUT index(1-60)"=w14759) -> ("DUT SC"=w14757:bool)  [unwired: 7 in, 3 out]
        n6913 = property class="ColBox"(reference=w14761, "Value"=u32 10000536 ("DRV 1")) -> ()  [unwired: 1 in, 2 out]
        n6914 = case shown="False" w14757 {
          tunnel: w14759 -> [w14777 _]
          tunnel: [w14776 w14842] -> w14758
          tunnel: w14756 -> [w14775 _]
          frame False {
            n6915 = case shown="True" w14775 {
              tunnel: w14777 -> [w14784 w14814]
              tunnel: [w14795 w14813] -> w14776
              frame False {
                w14781 = T9 {"command"="", "data"=variant} ("element")
                w14794 = T9 {"command"="", "data"=variant} ("element")
                n6916 = To Variant(anything=T3."mux10_1_channel9" ("mux10_1(x6)_encode")) -> (Variant=w14792:variant)
                n6917 = To Variant(anything=T4."demux1_10_channel9" ("demux1_10(x6)_encode")) -> (Variant=w14788:variant)
                n6918 = To Variant(anything=bool[] [FALSE, TRUE, FALSE, FALSE, FALSE, FALSE]) -> (Variant=w14803:variant)
                n6919 = Bundle By Name(cluster=w14794, "command"="MEAS.AllRelaysOFF") -> (w14802:T9)
                n6920 = Bundle By Name(cluster=w14794, "command"="MEAS.mux10-1", "data"=w14792) -> (w14785:T9)
                n6921 = Bundle By Name(cluster=w14794, "command"="MEAS.demux1-10", "data"=w14788) -> (w14786:T9)
                n6922 = Bundle By Name(cluster=w14794, "command"="MEAS.eMIC", "data"=w14803) -> (w14787:T9)
                n6923 = Build Array(w14802, w14785, w14786, w14787) -> (w14780:T9[])
                n6924 = To Variant(anything=w14784) -> (Variant=w14783:variant)
                n6925 = To Variant(anything=w14784) -> (Variant=w14782:variant)
                n6926 = Bundle By Name(cluster=w14781, "command"="MEAS.requestAC", "data"=w14783) -> (w14800:T9)
                n6927 = Bundle By Name(cluster=w14781, "command"="Apps.WaitForEvent", "data"=w14782) -> (w14796:T9)
                n6928 = Bundle By Name(cluster=w14781, "command"="Apps.UI Update 1") -> (w14797:T9)
                n6929 = Bundle By Name(cluster=w14781, "command"="WaitFor") -> (w14779:T9)
                n6930 = Build Array (concatenate)(w14780, w14779, w14800, w14796, w14797) -> (w14795:T9[])
              }
              frame True {
                w14810 = T9 {"command"="", "data"=variant} ("element")
                w14832 = T9 {"command"="", "data"=variant} ("element")
                n6931 = To Variant(anything=T3."mux10_1_channel9" ("mux10_1(x6)_encode")) -> (Variant=w14839:variant)
                n6932 = To Variant(anything=T2."mux6_1_channel2_3" ("mux6_1(3wires)_encode")) -> (Variant=w14837:variant)
                n6933 = To Variant(anything=T4."demux1_10_channel9" ("demux1_10(x6)_encode")) -> (Variant=w14833:variant)
                n6934 = To Variant(anything=bool[] [FALSE, TRUE, FALSE, FALSE, FALSE, FALSE]) -> (Variant=w14829:variant)
                n6935 = Bundle By Name(cluster=w14832, "command"="MEAS.AllRelaysOFF") -> (w14828:T9)
                n6936 = Bundle By Name(cluster=w14832, "command"="MEAS.mux10-1", "data"=w14839) -> (w14827:T9)
                n6937 = Bundle By Name(cluster=w14832, "command"="MEAS.mux6_1", "data"=w14837) -> (w14826:T9)
                n6938 = Bundle By Name(cluster=w14832, "command"="MEAS.demux1-10", "data"=w14833) -> (w14825:T9)
                n6939 = Bundle By Name(cluster=w14832, "command"="MEAS.eMIC", "data"=w14829) -> (w14824:T9)
                n6940 = Build Array(w14828, w14827, w14826, w14825, w14824) -> (w14809:T9[])
                n6941 = To Variant(anything=w14814) -> (Variant=w14812:variant)
                n6942 = To Variant(anything=w14814) -> (Variant=w14811:variant)
                n6943 = Bundle By Name(cluster=w14810, "command"="WaitFor") -> (w14808:T9)
                n6944 = Bundle By Name(cluster=w14810, "command"="MEAS.DMM dual read") -> (w14821:T9)
                n6945 = Bundle By Name(cluster=w14810, "command"="MEAS.requestAC", "data"=w14812) -> (w14820:T9)
                n6946 = Bundle By Name(cluster=w14810, "command"="Apps.WaitForEvent", "data"=w14811) -> (w14815:T9)
                n6947 = Bundle By Name(cluster=w14810, "command"="Apps.UI Update 1") -> (w14816:T9)
                n6948 = Build Array (concatenate)(w14809, w14808, w14821, w14820, w14815, w14816) -> (w14813:T9[])
              }
            }
          }
          frame True {
            n6949 = Bundle By Name(cluster=T9 {"command"="", "data"=variant} ("element"), "command"="Apps.UI Update 1") -> (w14843:T9)
            n6950 = Build Array(w14843) -> (w14842:T9[])
          }
        }
        n6951 = for {
          tunnel: w14758 -> [w14853] mode=indexing
          tunnel: w14766 -> [w14854]
          tunnel: [w14850] -> w14768 mode=indexing
          n6952 = Unbundle By Name(w14853) -> ("command"=w14852:string, "data"=w14851:variant)
          n6953 = call "App enquece.vi"("command data"=w14851, "command"=w14852, "queue in"=w14854) -> ("error out"=w14850:errorcluster)  [unwired: 7 in, 1 out]
        }
        n6954 = Merge Errors(w14769, w14768) -> (w14767:errorcluster)
      }
      frame "Test DRV 51A" {
        w14858 = 51 ("DUT index(0-59)")
        n6955 = disable-structure shown="LOGGING==TRUE" {
          disable-tunnel: w14863 -> [w14946 _]
          frame condition #0 (active) {
            n6956 = Empty String/Path?(string/path=w14946) -> (empty?=w14948:bool)
            n6957 = Select(t="Quece timeout", s=w14948, f=w14946) -> (s? t:f=w14945:string)
            n6958 = call "string log (SubVI).vi"("state Name"=w14945) -> ()  [unwired: 9 in, 2 out]
          }
          frame condition #1 {
          }
        }
        n6959 = Flush Queue(queue=w14864) -> (queue out=w14865:refnum<queue>)  [unwired: 1 in, 2 out]
        n6960 = Decrement(x=w14858) -> (x-1=w14862:i32)
        n6961 = Index Array(array=w14859, index=w14862) -> (element=w14860:refnum<vi>)
        n6962 = call "FGV DRV stand.vi"() -> ("Sub-Test.DCV"=w14855:bool)  [unwired: 10 in, 1 out]
        n6963 = call "FGV Driver Data.vi"("DUT index(1-60)"=w14858) -> ("DUT SC"=w14856:bool)  [unwired: 7 in, 3 out]
        n6964 = property class="ColBox"(reference=w14860, "Value"=u32 10000536 ("DRV 1")) -> ()  [unwired: 1 in, 2 out]
        n6965 = case shown="False" w14856 {
          tunnel: w14858 -> [w14876 _]
          tunnel: [w14875 w14941] -> w14857
          tunnel: w14855 -> [w14874 _]
          frame False {
            n6966 = case shown="False" w14874 {
              tunnel: w14876 -> [w14883 w14913]
              tunnel: [w14894 w14912] -> w14875
              frame False {
                w14880 = T9 {"command"="", "data"=variant} ("element")
                w14893 = T9 {"command"="", "data"=variant} ("element")
                n6967 = To Variant(anything=T3."mux10_1_channel9" ("mux10_1(x6)_encode")) -> (Variant=w14891:variant)
                n6968 = To Variant(anything=T4."demux1_10_channel9" ("demux1_10(x6)_encode")) -> (Variant=w14887:variant)
                n6969 = To Variant(anything=bool[] [FALSE, FALSE, TRUE, FALSE, FALSE, FALSE]) -> (Variant=w14902:variant)
                n6970 = Bundle By Name(cluster=w14893, "command"="MEAS.AllRelaysOFF") -> (w14901:T9)
                n6971 = Bundle By Name(cluster=w14893, "command"="MEAS.mux10-1", "data"=w14891) -> (w14884:T9)
                n6972 = Bundle By Name(cluster=w14893, "command"="MEAS.demux1-10", "data"=w14887) -> (w14885:T9)
                n6973 = Bundle By Name(cluster=w14893, "command"="MEAS.eMIC", "data"=w14902) -> (w14886:T9)
                n6974 = Build Array(w14901, w14884, w14885, w14886) -> (w14879:T9[])
                n6975 = To Variant(anything=w14883) -> (Variant=w14882:variant)
                n6976 = To Variant(anything=w14883) -> (Variant=w14881:variant)
                n6977 = Bundle By Name(cluster=w14880, "command"="MEAS.requestAC", "data"=w14882) -> (w14899:T9)
                n6978 = Bundle By Name(cluster=w14880, "command"="Apps.WaitForEvent", "data"=w14881) -> (w14895:T9)
                n6979 = Bundle By Name(cluster=w14880, "command"="Apps.UI Update 1") -> (w14896:T9)
                n6980 = Bundle By Name(cluster=w14880, "command"="WaitFor") -> (w14878:T9)
                n6981 = Build Array (concatenate)(w14879, w14878, w14899, w14895, w14896) -> (w14894:T9[])
              }
              frame True {
                w14909 = T9 {"command"="", "data"=variant} ("element")
                w14931 = T9 {"command"="", "data"=variant} ("element")
                n6982 = To Variant(anything=T3."mux10_1_channel9" ("mux10_1(x6)_encode")) -> (Variant=w14938:variant)
                n6983 = To Variant(anything=T2."mux6_1_channel3_3" ("mux6_1(3wires)_encode")) -> (Variant=w14936:variant)
                n6984 = To Variant(anything=T4."demux1_10_channel9" ("demux1_10(x6)_encode")) -> (Variant=w14932:variant)
